vi "Configure External Control.vi"(5 "Output Control Logic (0: LowEnablesOutput)":i32(ring) items=["Low Enables Output", "High Enables Output"], 6 "Control Range (0: Low)":i32(ring) items=["Low", "High"], 7 "Enable External Output Control (F: Disable)":bool, 8 "error in (no error)":errorcluster, 9 "Enable External Voltage Control (F: Disable)":bool, 10 "Enable External Current Control (F: Disable)":bool, 11 "VISA resource name":refnum<visa-resource-name>) -> (0 "error out":errorcluster, 3 "VISA resource name out":refnum<visa-resource-name>)   [LabVIEW 2023]
doc: "Configures external control settings."
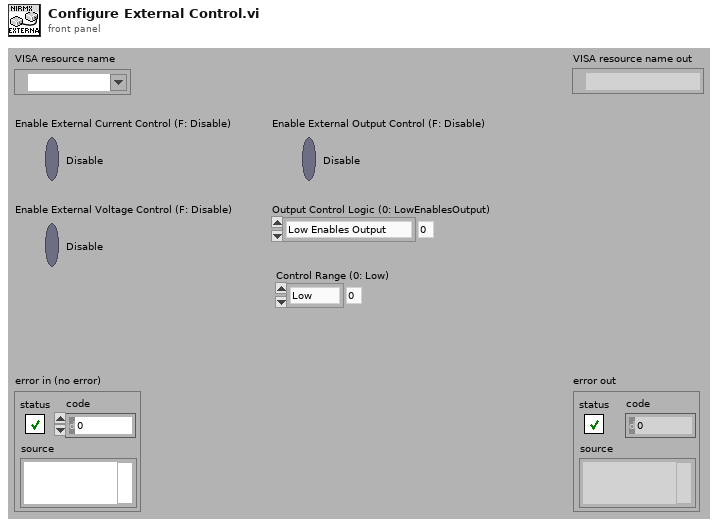
[diagram p1: front panel]
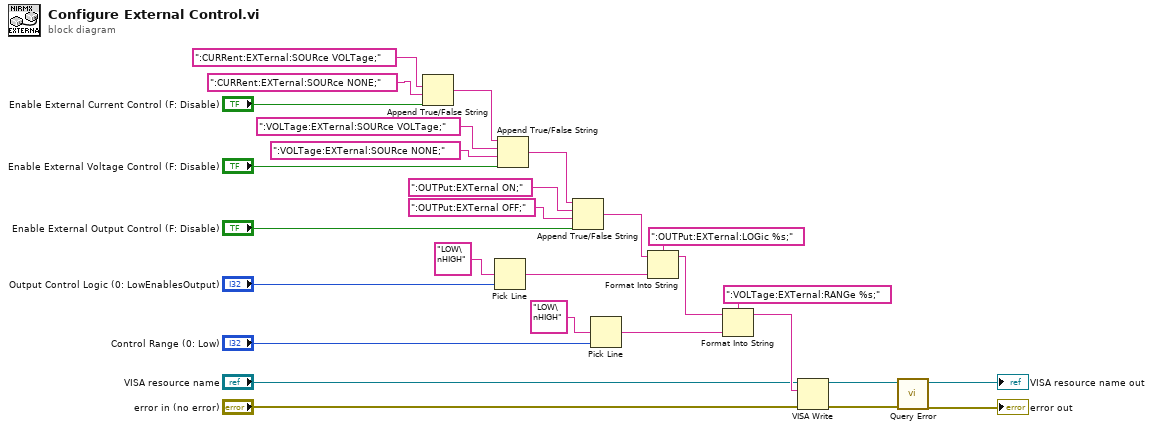
[diagram p0: block diagram]
diagram:
  n1 = Append True/False String(1:"Enable External Current Control (F: Disable)", 2:":CURRent:EXTernal:SOURce NONE;", 3:":CURRent:EXTernal:SOURce VOLTage;") -> (0:w27:string)  [unwired: 1 in]
  n2 = Pick Line(multi-line string="LOW\nHIGH", line index="Output Control Logic (0: LowEnablesOutput)") -> (output string=w9:string)  [unwired: 1 in]
  n3 = Append True/False String(1:"Enable External Voltage Control (F: Disable)", 2:":VOLTage:EXTernal:SOURce NONE;", 3:":VOLTage:EXTernal:SOURce VOLTage;", 4:w27) -> (0:w25:string)
  n4 = Append True/False String(1:"Enable External Output Control (F: Disable)", 2:":OUTPut:EXTernal OFF;", 3:":OUTPut:EXTernal ON;", 4:w25) -> (0:w21:string)
  n5 = Pick Line(multi-line string="LOW\nHIGH", line index="Control Range (0: Low)") -> (output string=w6:string)  [unwired: 1 in]
  n6 = Format Into String(format string=":OUTPut:EXTernal:LOGic %s;", initial string=w21, w9) -> (resulting string=w19:string)  [unwired: 1 in, 1 out]
  n7 = Format Into String(format string=":VOLTage:EXTernal:RANGe %s;", initial string=w19, w6) -> (resulting string=w17:string)  [unwired: 1 in, 1 out]
  n8 = VISA Write(VISA resource name="VISA resource name", write buffer=w17, error in (no error)="error in (no error)") -> (VISA resource name out=w14:refnum<visa-resource-name>, error out=w13:errorcluster)  [unwired: 1 out]
  n9 = call "Query Error.vi"("error in (no error)"=w13, "VISA resource name"=w14) -> ("error out"=→"error out":errorcluster, "VISA resource name out"=→"VISA resource name out":refnum<visa-resource-name>)  [unwired: 6 in, 2 out]
